vi "Configure FGEN.vi"(8 "error in":errorcluster, 9 "Waveforms":waveform(dbl)[](array[waveform]), 10 "FGEN Session":refnum<k15>, 11 "measurement configuration in":T1) -> (0 "error out":errorcluster, 1 "Actual Sample Rate":dbl, 2 "FGEN Session Out":refnum<k15>, 3 "measurement configuration out":T1)   [LabVIEW 2025, in "Fgen Script Mode.lvclass"]
uses:
  Fgen Script Mode.lvclass
  Fgen Script Mode.lvclass/Fgen Script Mode.ctl
  <instrlib>/niFgen/niFgen.llb/niFgen Output Mode.ctl
  Typedef/Trigger Settings.ctl
  <instrlib>/niFgen/niFgen.llb/niFgen_ctl Trigger Script - trigID Values (Ring).ctl
  <instrlib>/niFgen/niFgen.llb/niFgen Write Named Waveform (WDT).vi
  <instrlib>/niFgen/niFgen.llb/niFgen_ctl Exported Signal Identifiers (Ring).ctl
  <instrlib>/niFgen/niFgen.llb/niFgen_ctl Exported Signal Name Values (Ring).ctl
  <instrlib>/niFgen/niFgen.llb/niFgen Configure Digital Edge Script Trigger.vi
  Measurement Configuration.ctl
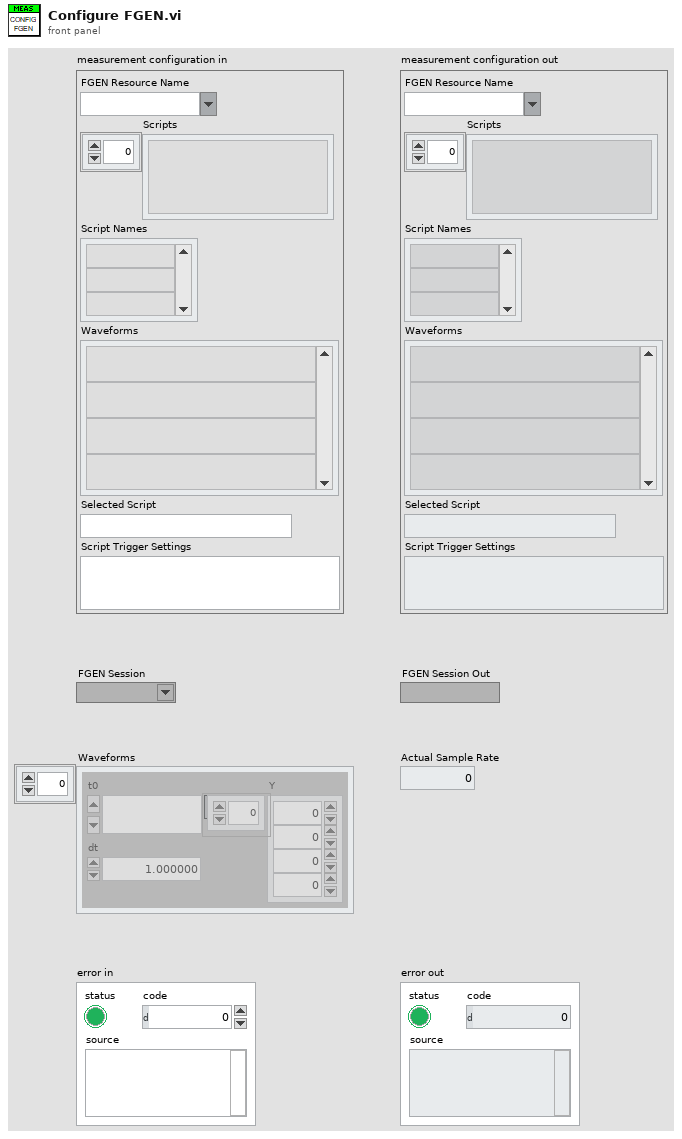
[diagram p1: front panel]
types:
  T1 = typedef "Fgen Script Mode.lvclass/Measurement Configuration.ctl" = cluster{"FGEN Resource Name":string, "Scripts":string[], "Script Names":string[], "Waveforms":string[], "Selected Script":string, "Script Trigger Settings":string}
  T2 = typedef "niFgen_ctl Exported Signal Identifiers (Ring).ctl" = string
  T3 = typedef "niFgen_ctl Trigger Script - trigID Values (Ring).ctl" = string
  T4 = typedef "Fgen Script Mode.lvclass/Trigger Settings.ctl" = cluster{"Script Trigger 0 Source":string, "Script Trigger 1 Source":string, "Script Trigger 2 Source":string, "Script Trigger 3 Source":string, "Marker0 Output Terminal":string, "Marker1 Output Terminal":string, "Marker2 Output Terminal":string, "Marker3 Output Terminal":string}
  T5 = typedef "niFgen Output Mode.ctl" = u32
  T6 = typedef "niFgen_ctl Exported Signal Name Values (Ring).ctl" = u16
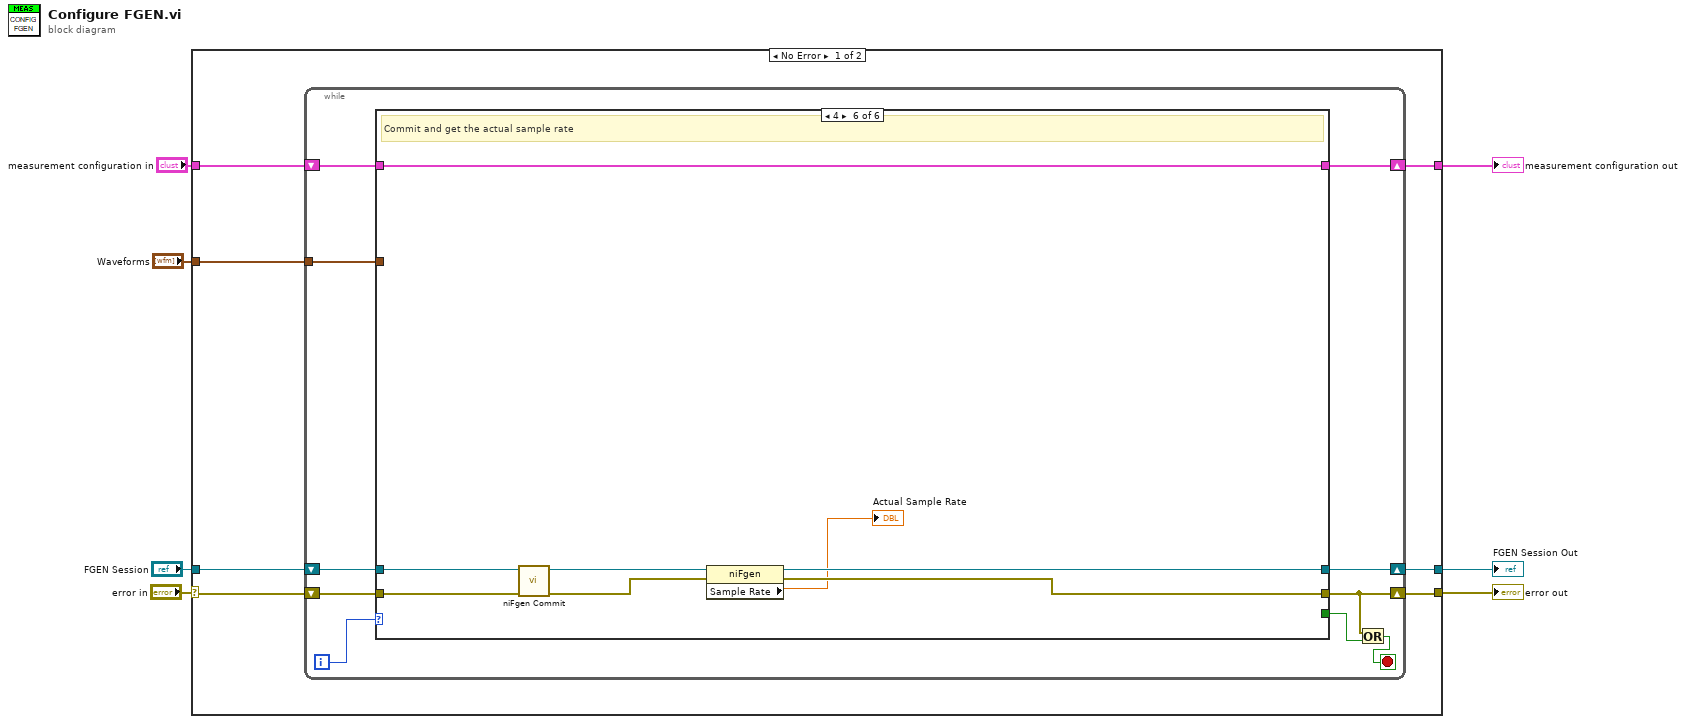
[diagram p0: block diagram]
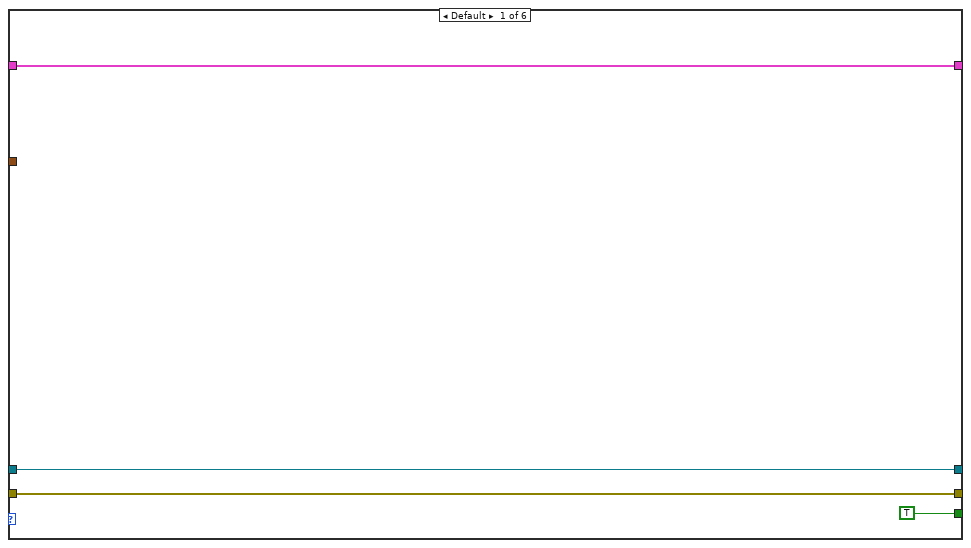
[diagram p2: hidden frame]
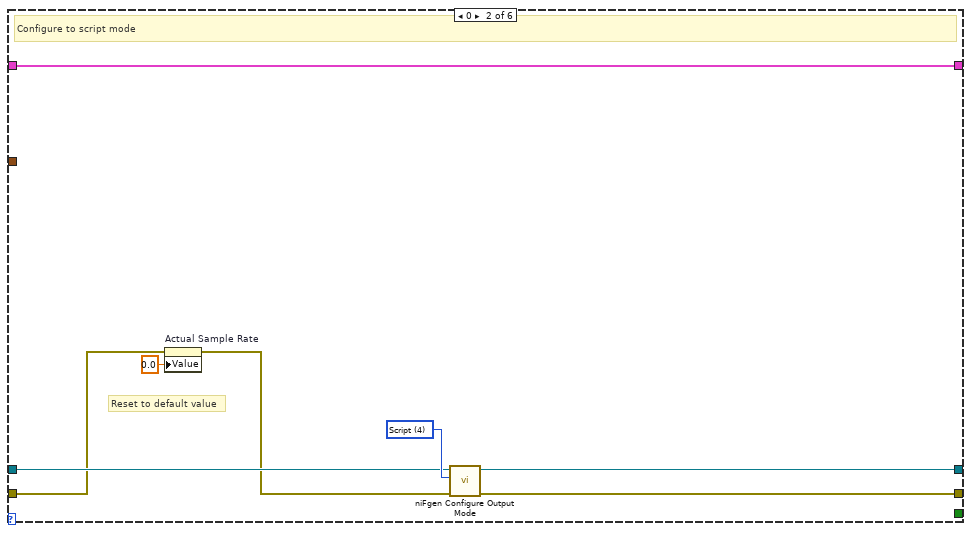
[diagram p3: hidden frame]
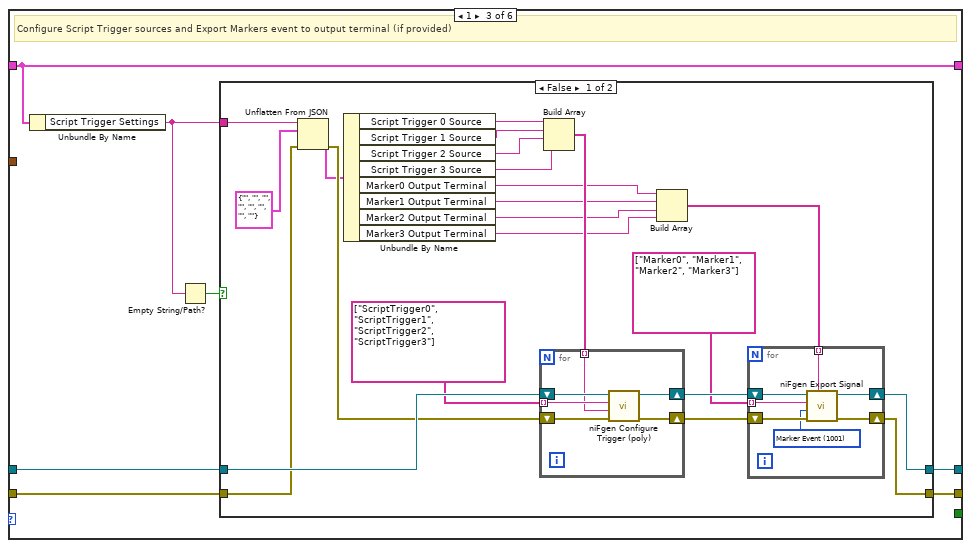
[diagram p4: hidden frame]
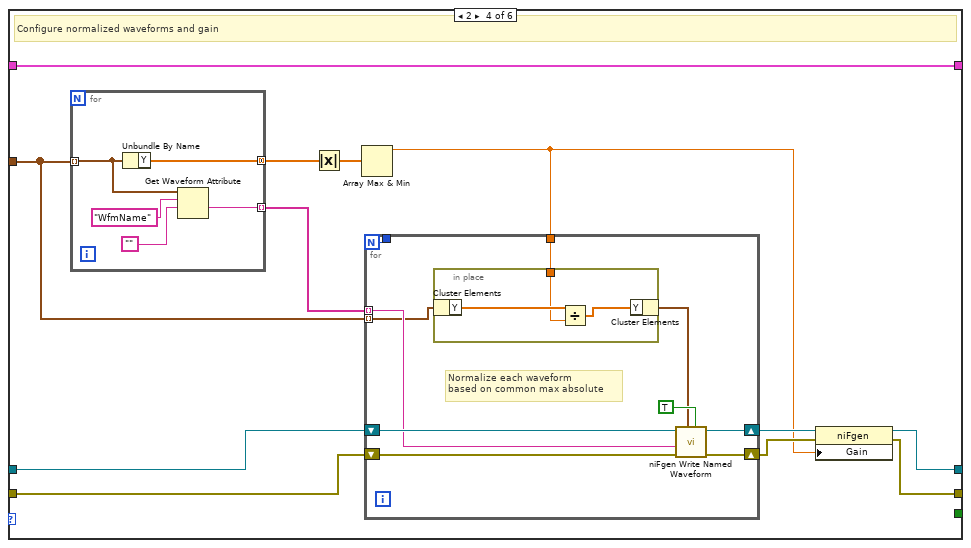
[diagram p6: hidden frame]
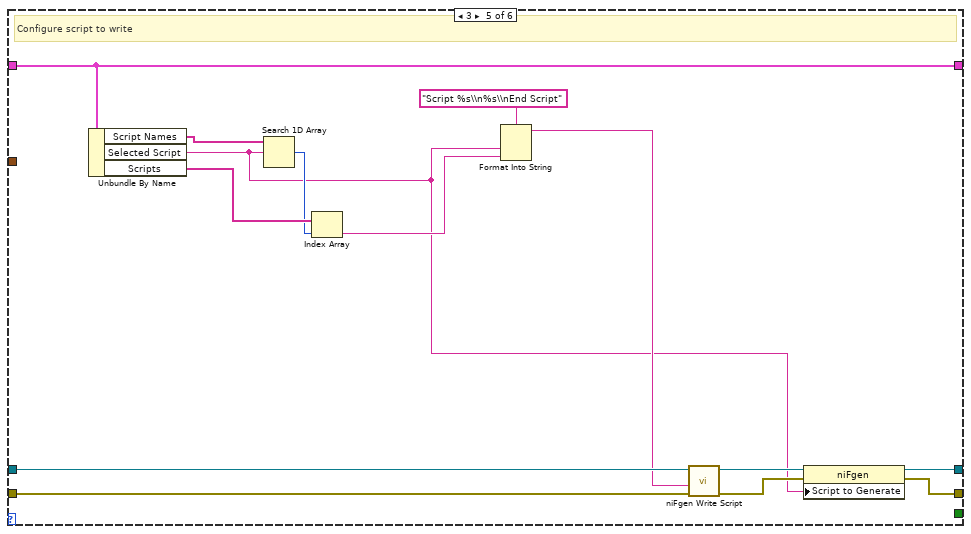
[diagram p7: hidden frame]
diagram:
  n1 = case shown="No Error" "error in" {
    selector: "error in" -> [w11 w135]
    tunnel: [w12 w135] -> w6
    tunnel: "measurement configuration in" -> [w14 w134]
    tunnel: [w13 w134] -> w4
    tunnel: "Waveforms" -> [w10 _]
    tunnel: "FGEN Session" -> [w9 w133]
    tunnel: [w8 w133] -> w1
    frame No Error {
      n2 = while {
        shift-right: [w22] -> w13
        shift-left: w14 -> [w23]
        shift-right: [w17] -> w12
        shift-left: w11 -> [w21]
        tunnel: w10 -> [w20]
        shift-right: [w19] -> w8
        shift-left: w9 -> [w18]
        i -> [w24]
        stop <- w16 stop-if-true
        n3 = case shown="4" w24 {
          tunnel: w23 -> [w28 w36 w42 w92 w121 w132]
          tunnel: [w28 w36 w42 w92 w121 w132] -> w22
          tunnel: [w27 w32 w40 w82 w114 w128] -> w17
          tunnel: w21 -> [w27 w30 w41 w86 w124 w131]
          tunnel: w20 -> [_ _ _ w89 _ _]
          tunnel: [w26 w34 w39 w81 w112 w126] -> w19
          tunnel: w18 -> [w26 w33 w43 w87 w122 w129]
          tunnel: [TRUE _ _ _ _ _] -> w15
          frame Default {
          }
          frame 0 {
            w35 = T5 4 items=["Standard Function", "Frequency List", "Arbitrary Waveform", "Arbitrary Sequence", "Script"] ("Output Mode")
            # "Reset to default value"
            # "Configure to script mode"
            n4 = property on="Actual Sample Rate" class="DigNum (strict)"(error in=w30, "Value"=0.0 ("Actual Sample Rate")) -> (error out=w29:errorcluster)  [unwired: 1 in, 1 out]
            n5 = call <instrlib>:"niFgen Configure Output Mode.vi"("error in (no error)"=w29, "Output Mode (default: 0=Standard Function)"=w35, "Instrument Handle"=w33) -> ("error out"=w32:errorcluster, "Instrument Handle Out"=w34:refnum<k15>)  [unwired: 6 in]
          }
          frame 1 {
            # "Configure Script Trigger sources and Export Markers event to output terminal (if provided)"
            n6 = Unbundle By Name(w42) -> ("Script Trigger Settings"=w37:string)
            n7 = Empty String/Path?(string/path=w37) -> (empty?=w38:bool)
            n8 = case shown="False" w38 {
              tunnel: w43 -> [w64 w80]
              tunnel: w37 -> [w63 _]
              tunnel: w41 -> [w61 w79]
              tunnel: [w52 w79] -> w40
              tunnel: [w50 w80] -> w39
              frame False {
                n9 = Unflatten From JSON(JSON string=w63, type and defaults=T4 {"Script Trigger 0 Source"="", "Script Trigger 1 Source"="", "Script Trigger 2 Source"="", "Script Trigger 3 Source"="", "Marker0 Output Terminal"="", "Marker1 Output Terminal"="", "Marker2 Output Terminal"="", "Marker3 Output Terminal"=""} ("Trigger Settings"), error in (no error)=w61) -> (value=w59:T4, error out=w60:errorcluster)  [unwired: 4 in]
                n10 = Unbundle By Name(w59) -> ("Script Trigger 0 Source"=w57:string, "Script Trigger 1 Source"=w56:string, "Script Trigger 2 Source"=w53:string, "Script Trigger 3 Source"=w55:string, "Marker0 Output Terminal"=w48:string, "Marker1 Output Terminal"=w47:string, "Marker2 Output Terminal"=w46:string, "Marker3 Output Terminal"=w45:string)
                n11 = Build Array(w57, w56, w53, w55) -> (w54:string[])
                n12 = for {
                  tunnel: T3[] ["ScriptTrigger0", "ScriptTrigger1", "ScriptTrigger2", "ScriptTrigger3"] ("Array") -> [w74] mode=indexing
                  shift-right: [w76] -> w51
                  shift-left: w64 -> [w77]
                  shift-right: [w78] -> w65
                  shift-left: w60 -> [w75]
                  tunnel: w54 -> [w73] mode=indexing
                  n13 = call-poly <instrlib>:"niFgen Configure Trigger (poly).vi"("error in (no error)"=w75, "Source"=w73, "Trigger ID (Script Trigger 0)"=w74, "Instrument Handle"=w77) -> ("error out"=w78:errorcluster, "Instrument Handle Out"=w76:refnum<k15>)  [unwired: 6 in]
                }
                n14 = Build Array(w48, w47, w46, w45) -> (w44:string[])
                n15 = for {
                  shift-right: [w71] -> w52
                  shift-left: w65 -> [w72]
                  shift-right: [w69] -> w50
                  shift-left: w51 -> [w70]
                  tunnel: T2[] ["Marker0", "Marker1", "Marker2", "Marker3"] ("Array") -> [w68] mode=indexing
                  tunnel: w44 -> [w67] mode=indexing
                  w66 = T6 1001 items=["Sample Clock"=101, "Sample Clock Timebase"=1006, "Reference Clock"=102, "Onboard Reference Clock"=1019, "Start Trigger"=1004, "Script Trigger"=103, "Marker Event"=1001, "Data Marker Event"=108, "Ready For Start Event"=105, "Started Event"=106, "Done Event"=107, "Synchronization Pulse"=1007, "Sync Out"=1002] ("Signal")
                  n16 = call <instrlib>:"niFgen Export Signal.vi"("Output Terminal (do not export)"=w67, "error in (no error)"=w72, "Signal"=w66, "Signal Identifier (None)"=w68, "Instrument Handle"=w70) -> ("error out"=w71:errorcluster, "Instrument Handle Out"=w69:refnum<k15>)  [unwired: 5 in]
                }
              }
              frame True {
              }
            }
          }
          frame 2 {
            # "Configure normalized waveforms and gain"
            n17 = for {
              tunnel: w89 -> [w110] mode=indexing
              tunnel: [w108] -> w88 mode=indexing
              tunnel: [w106] -> w91 mode=concatenating
              n18 = Unbundle By Name(w110) -> ("Y"=w106:dbl[])
              n19 = Get Waveform Attribute(5:"", 6:"WfmName" ("name"), 7:w110) -> (1:w108:string)  [unwired: 1 in, 3 out]
            }
            n20 = Absolute Value(x=w91) -> (abs(x)=w90:dbl[])
            n21 = Array Max & Min(array=w90) -> (max value=w83:dbl)  [unwired: 3 out]
            n22 = for {
              N -> [w96]
              shift-right: [w102] -> w84
              shift-left: w86 -> [w101]
              tunnel: w89 -> [w95] mode=indexing
              tunnel: w88 -> [w99] mode=indexing
              shift-right: [w97] -> w85
              shift-left: w87 -> [w100]
              tunnel: [w96] -> _
              tunnel: w83 -> [w93]
              # "Normalize each waveform\nbased on common max absolute"
              n23 = in-place {
                in-place-border: w93 -> [w103]
                n24 = in-place-cluster #1(w95) -> ("Y"=w105:dbl[])
                n25 = Divide(x=w105, y=w103) -> (x/y=w104:dbl[])
                n26 = in-place-cluster #1("Y"=w104) -> (w94:waveform(dbl))
              }
              n27 = call-poly <instrlib>:"niFgen Write Named Waveform.vi"("Use Waveform dT for Sample Rate"=TRUE, "Waveform"=w94, "error in (no error)"=w101, "Waveform Name"=w99, "Instrument Handle"=w100) -> ("error out"=w102:errorcluster, "Instrument Handle Out"=w97:refnum<k15>)  [unwired: 4 in, 1 out]
            }
            n28 = property class="niFgen"(reference=w85, error in=w84, "Gain"=w83) -> (reference out=w81:refnum<k15>, error out=w82:errorcluster)
          }
          frame 3 {
            # "Configure script to write"
            n29 = Unbundle By Name(w121) -> ("Script Names"=w119:string[], "Selected Script"=w111:string, "Scripts"=w118:string[])
            n30 = Search 1D Array(1D array=w119, element=w111) -> (index of element=w117:i32)  [unwired: 1 in]
            n31 = Index Array(array=w118, index=w117) -> (element=w116:string)
            n32 = Format Into String(format string="Script %s\\n%s\\nEnd Script", w111, w116) -> (resulting string=w115:string)  [unwired: 2 in, 1 out]
            n33 = call <instrlib>:"niFgen Write Script.vi"("error in (no error)"=w124, "Script"=w115, "Instrument Handle"=w122) -> ("error out"=w123:errorcluster, "Instrument Handle Out"=w113:refnum<k15>)  [unwired: 7 in]
            n34 = property class="niFgen"(reference=w113, error in=w123, "Script to Generate"=w111) -> (reference out=w112:refnum<k15>, error out=w114:errorcluster)
          }
          frame 4 {
            # "Commit and get the actual sample rate"
            n35 = call <instrlib>:"niFgen Commit.vi"("error in (no error)"=w131, "Instrument Handle"=w129) -> ("error out"=w130:errorcluster, "Instrument Handle Out"=w127:refnum<k15>)  [unwired: 8 in]
            n36 = property class="niFgen"(reference=w127, error in=w130) -> (reference out=w126:refnum<k15>, error out=w128:errorcluster, "Sample Rate"=→"Actual Sample Rate":dbl)
          }
        }
        n37 = Or(x=w17, y=w15) -> (x .or. y?=w16:bool)
      }
    }
    frame Error {
    }
  }
  "measurement configuration out" <- w4
  "error out" <- w6
  "FGEN Session Out" <- w1
